vi "nodeInfo.VI-Tree.vi"() -> ()   [LabVIEW 2014, in "LVNodeInfo.lvlib"]
doc: "VI Tree for a a library, that allows to obtain information about the local node."
uses:
  LVNodeInfo.lvlib
panel:
  out "error out":errorcluster
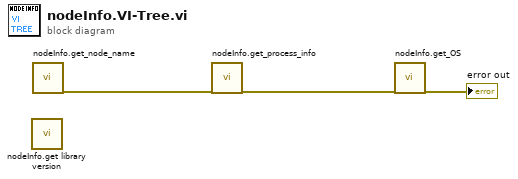
[diagram p0: block diagram]
diagram:
  n1 = call "nodeInfo.get library version.vi"() -> ()  [unwired: 1 in, 1 out]
  n2 = call "nodeInfo.get_node_name.vi"() -> ("error out"=w3:errorcluster)  [unwired: 18 in, 1 out]
  n3 = call "nodeInfo.get_process_info.vi"("error in (no error)"=w3) -> ("error out"=w2:errorcluster)  [unwired: 13 in, 5 out]
  n4 = call "nodeInfo.get_OS.vi"("error in (no error)"=w2) -> ("error out"=→"error out":errorcluster)  [unwired: 17 in, 1 out]
